vi "TempMeas.vi"   [LabVIEW 2015]
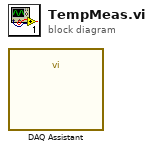
[diagram p0: block diagram]
diagram:
  n1 = call "DAQ Assistant"() -> ()  [unwired: 17 in, 3 out]
